vi "CheckForSMax.vi"(8 "error in (no error)":errorcluster, 10 "chanel in":T1) -> (0 "error out":errorcluster, 2 "chanel out":T1, 3 "contains smax":bool)   [LabVIEW 2017, in "AnalysisHelper.lvlib"]
uses:
  <vilib>/addons/InsightCM/Utilities/Analysis/Shared/AnalysisHelper.lvlib
  <vilib>/addons/InsightCM/Utilities/Analysis/Shared/controls/Channel.ctl
  <vilib>/addons/InsightCM/Utilities/Analysis/Shared/controls/SpeedType.ctl
  <vilib>/addons/InsightCM/Utilities/Analysis/Shared/controls/Feature.ctl
  <vilib>/addons/InsightCM/Utilities/Analysis/Shared/controls/AmplitudeScale.ctl
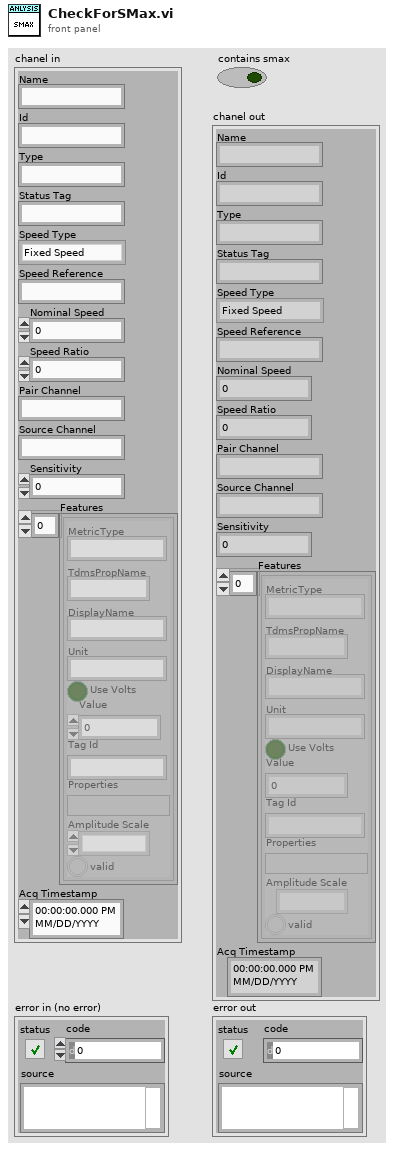
[diagram p1: front panel]
types:
  T1 = typedef "AnalysisHelper.lvlib/Channel.ctl" = cluster{"Name":string, "Id":string, "Type":string, "Status Tag":string, "Speed Type":T2, "Speed Reference":string, "Nominal Speed":dbl, "Speed Ratio":dbl, "Pair Channel":string, "Source Channel":string, "Sensitivity":dbl, "Features":T3[], "Acq Timestamp":timestamp}
  T2 = typedef "AnalysisHelper.lvlib/SpeedType.ctl" = enum16{"Fixed Speed", "Tachometer"}
  T3 = typedef "AnalysisHelper.lvlib/Feature.ctl" = cluster{"MetricType":string, "TdmsPropName":string, "DisplayName":string, "Unit":string, "Use Volts":bool, "Value":dbl, "Tag Id":string, "Properties":variant, "Amplitude Scale":T4, "valid":bool}
  T4 = typedef "AnalysisHelper.lvlib/AmplitudeScale.ctl" = enum16{"rms", "peak", "pk-pk"}
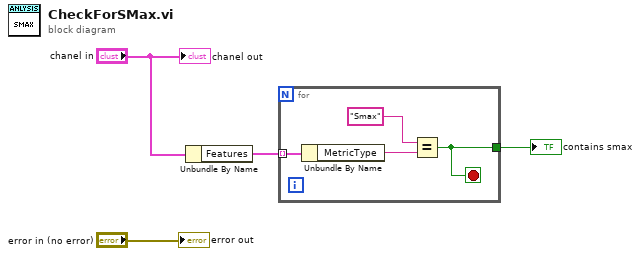
[diagram p0: block diagram]
diagram:
  n1 = Unbundle By Name("chanel in") -> ("Features"=w4:T3[])
  n2 = for {
    tunnel: w4 -> [w8] mode=indexing
    tunnel: [w5] -> w3
    stop <- w5 stop-if-true
    n3 = Unbundle By Name(w8) -> ("MetricType"=w7:string)
    n4 = Equal?(x="Smax", y=w7) -> (x = y?=w5:bool)
  }
  "contains smax" <- w3
  "error out" <- "error in (no error)"
  "chanel out" <- "chanel in"
